vi "Get Bounds.vi"(0 "Initial Time Bounds":dbl, 1 "Final Time Bounds":dbl, 2 "Initial State Bounds":dbl[][](array[numeric]), 3 "Final State Bounds":dbl[][](array[numeric]), 4 "Control Bounds":dbl[][](array[numeric]), 5 "State Bounds":dbl[][](array[numeric]), 6 "nGrid":dbl, 7 "Tolerance":dbl=0.01) -> (14 "bLow":dbl[](array[numeric]), 15 "bHigh":dbl[](array[numeric]))   [LabVIEW 2020]
uses:
  <vilib>/Analysis/1siggen.llb/Ramp Pattern by Samples.vi
  <vilib>/Analysis/NI_AALBase.lvlib
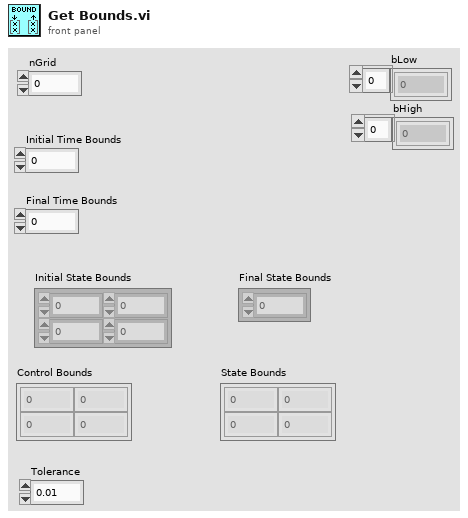
[diagram p1: front panel]
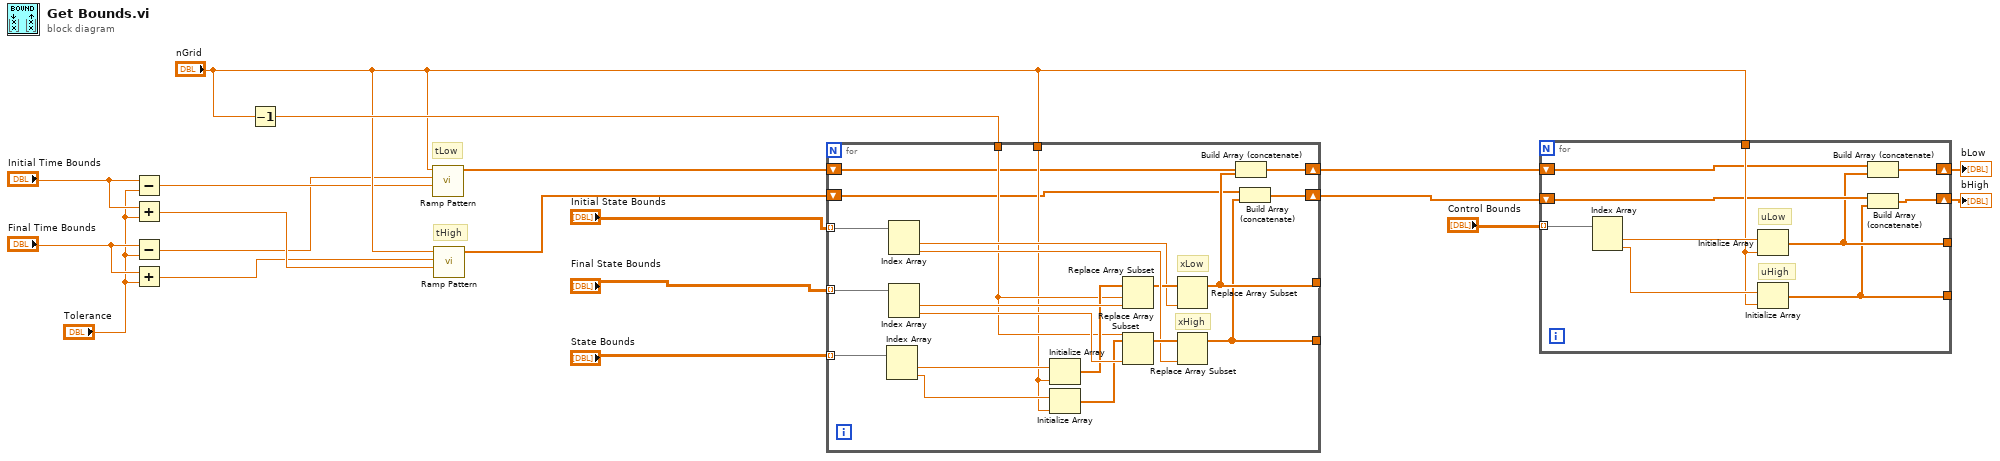
[diagram p0: block diagram]
diagram:
  # "tHigh"
  # "tLow"
  n1 = Subtract(x="Initial Time Bounds", y="Tolerance") -> (x-y=w7:dbl)
  n2 = Add(x="Initial Time Bounds", y="Tolerance") -> (x+y=w6:dbl)
  n3 = Subtract(x="Final Time Bounds", y="Tolerance") -> (x-y=w5:dbl)
  n4 = Add(x="Final Time Bounds", y="Tolerance") -> (x+y=w4:dbl)
  n5 = Decrement(x="nGrid") -> (x-1=w19:dbl)
  n6 = call-poly <vilib>:"Ramp Pattern.vi"("start"=w7, "end"=w5, "samples"="nGrid") -> ("Ramp Pattern"=w16:dbl[])  [unwired: 7 in, 1 out]
  n7 = call-poly <vilib>:"Ramp Pattern.vi"("start"=w6, "end"=w4, "samples"="nGrid") -> ("Ramp Pattern"=w15:dbl[])  [unwired: 7 in, 1 out]
  n8 = for {
    tunnel: [w21] -> _
    tunnel: [w23] -> _
    tunnel: w19 -> [w30]
    tunnel: "nGrid" -> [w29]
    tunnel: "Initial State Bounds" -> [w28] mode=indexing
    tunnel: "Final State Bounds" -> [w27] mode=indexing
    tunnel: "State Bounds" -> [w26] mode=indexing
    shift-right: [w25] -> w14
    shift-left: w16 -> [w24]
    shift-right: [w20] -> w13
    shift-left: w15 -> [w22]
    # "xHigh"
    # "xLow"
    n9 = Index Array(array=w26) -> (element #1=w31:dbl, element #2=w32:dbl)  [unwired: 2 in]
    n10 = Index Array(array=w28) -> (element #1=w35:dbl, element #2=w37:dbl)  [unwired: 2 in]
    n11 = Index Array(array=w27) -> (element #1=w34:dbl, element #2=w40:dbl)  [unwired: 2 in]
    n12 = Initialize Array(w31, w29) -> (w33:dbl[])
    n13 = Initialize Array(w32, w29) -> (w39:dbl[])
    n14 = Replace Array Subset(array=w33, new element=w34, index=w30) -> (w36:dbl[])
    n15 = Replace Array Subset(array=w39, new element=w40, index=w30) -> (w38:dbl[])
    n16 = Replace Array Subset(array=w36, new element=w35) -> (w23:dbl[])  [unwired: 1 in]
    n17 = Replace Array Subset(array=w38, new element=w37) -> (w21:dbl[])  [unwired: 1 in]
    n18 = Build Array (concatenate)(w24, w23) -> (w25:dbl[])
    n19 = Build Array (concatenate)(w22, w21) -> (w20:dbl[])
  }
  n20 = for {
    tunnel: [w43] -> _
    tunnel: [w44] -> _
    tunnel: "nGrid" -> [w48]
    tunnel: "Control Bounds" -> [w47] mode=indexing
    shift-right: [w42] -> w11
    shift-left: w14 -> [w46]
    shift-right: [w41] -> w10
    shift-left: w13 -> [w45]
    # "uHigh"
    # "uLow"
    n21 = Index Array(array=w47) -> (element #1=w49:dbl, element #2=w50:dbl)  [unwired: 2 in]
    n22 = Initialize Array(w49, w48) -> (w44:dbl[])
    n23 = Initialize Array(w50, w48) -> (w43:dbl[])
    n24 = Build Array (concatenate)(w46, w44) -> (w42:dbl[])
    n25 = Build Array (concatenate)(w45, w43) -> (w41:dbl[])
  }
  "bLow" <- w11
  "bHigh" <- w10
